vi "连接拧紧轴数据库.vi"(8 "error in (no error)":errorcluster, 9 "30":string="0", 10 "1":string="0", 11 "确定按钮":bool) -> (0 "error out":errorcluster, 1 "子数组":string[](array[string]), 2 "时间":string, 3 "索引结果":bool=TRUE)   [LabVIEW 2013]
uses:
  <vilib>/Utility/error.llb/whitespace.ctl
panel:
  out "error out 3":errorcluster
  out "error out 2":errorcluster
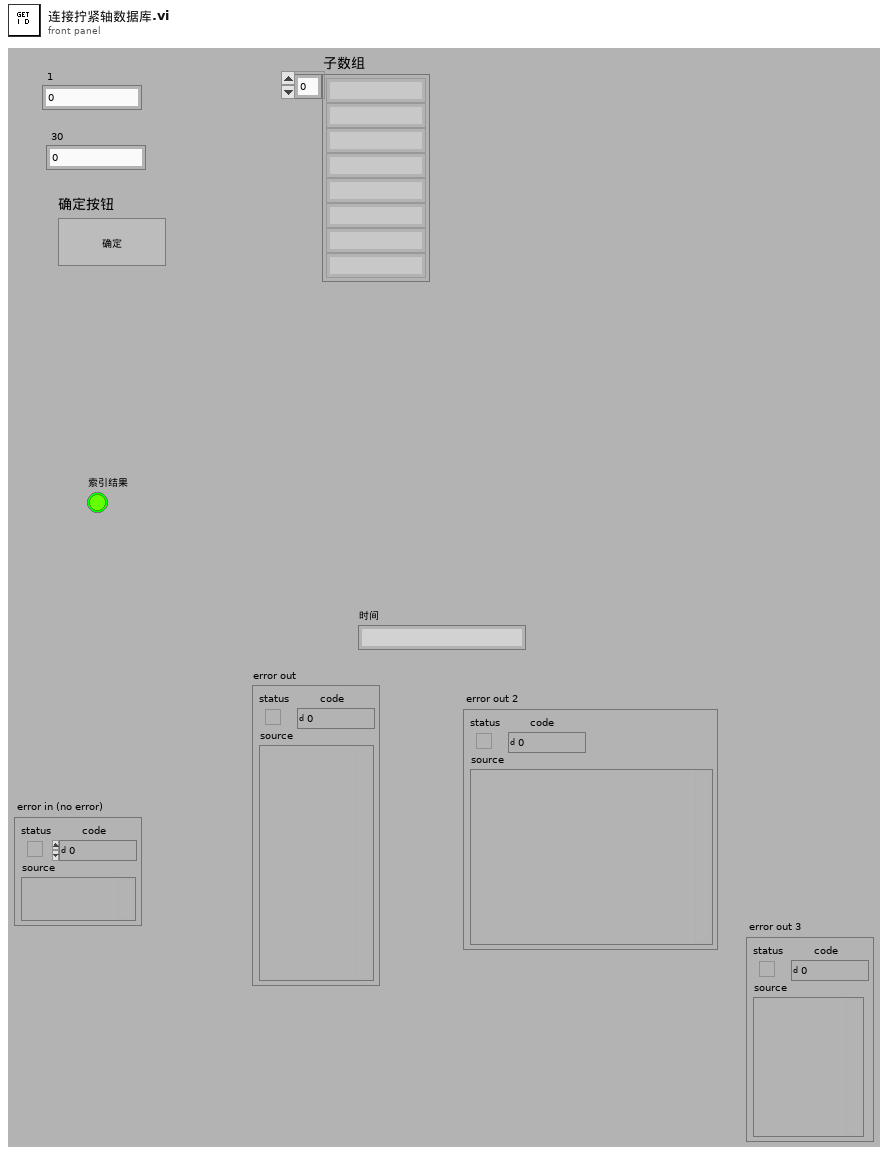
[diagram p1: front panel]
types:
  T1 = typedef "whitespace.ctl" = u16
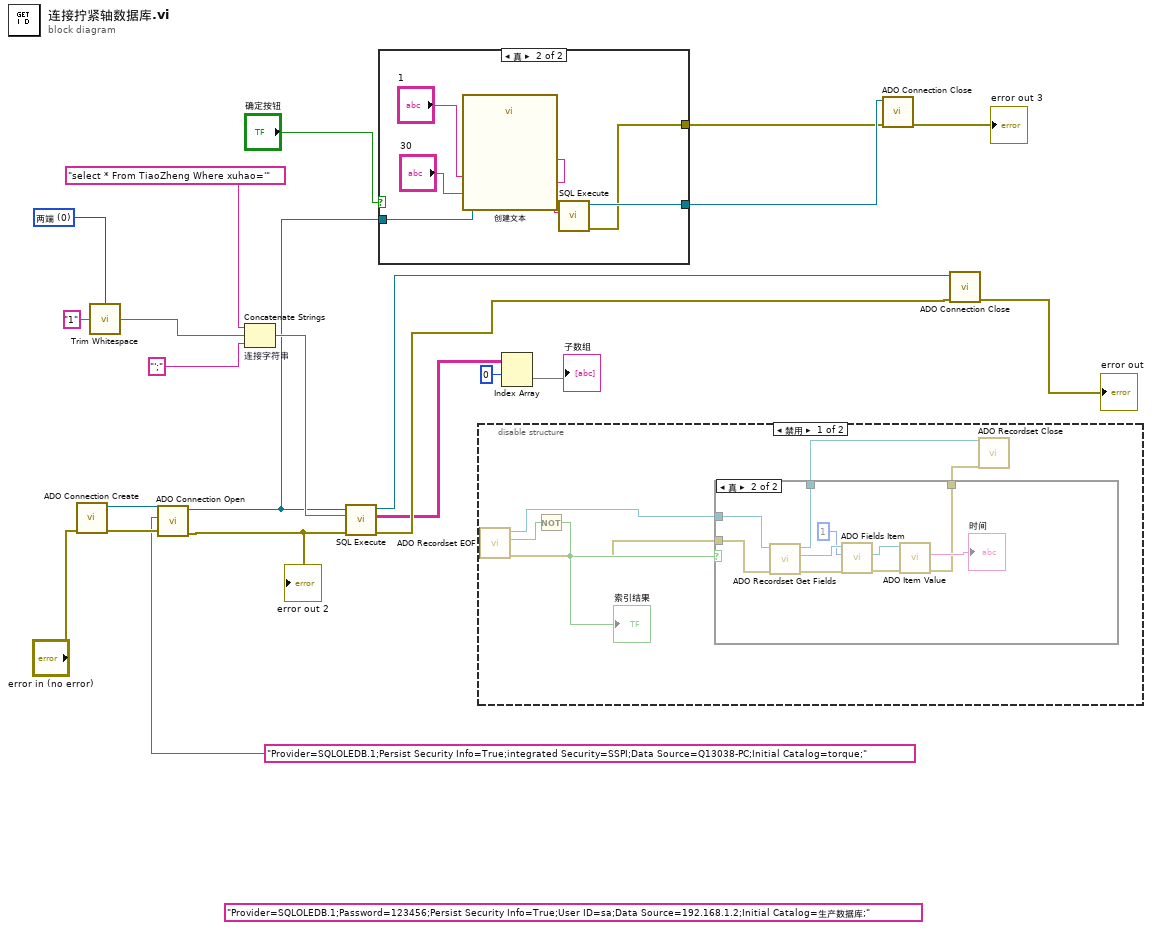
[diagram p0: block diagram]
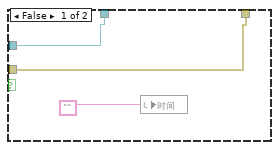
[diagram p3: hidden frame]
diagram:
  (unwired) "Provider=SQLOLEDB.1;Password=123456;Persist Security Info=True;User ID=sa;Data Source=192.168.1.2;Initial Catalog=生产数据库;" ("字符串 2")
  w15 = T1 0 items=["两端", "字符串首端", "字符串末端"] ("location (both)")
  n1 = call "ADO Connection Create.vi"("error in (no error)"="error in (no error)") -> ("error out"=w21:errorcluster, "ADODB._Connection Out"=w22:refnum<k7>)  [unwired: 9 out]
  n2 = call <vilib>:"Trim Whitespace.vi"("string"="1", "location (both)"=w15) -> ("trimmed string"=w16:string)
  n3 = call "ADO Connection Open.vi"("error in (no error)"=w21, "ConnectionString"="Provider=SQLOLEDB.1;Persist Security Info=True;integrated Security=SSPI;Data Source=Q13038-PC;Initial Catalog=torque;" ("字符串 2"), "ADODB._Connection In"=w22) -> ("error out"=w20:errorcluster, "ADODB._Connection Out"=w5:refnum<k7>)  [unwired: 7 out]
  "error out 2" <- w20
  n4 = Concatenate Strings "连接字符串"("select * From TiaoZheng Where xuhao='" ("字符串 2"), w16, "';" ("字符串 2")) -> (w6:string)
  n5 = call "SQL Execute.vi"("error in (no error)"=w20, "Command Text"=w6, "ADODB._Connection In"=w5) -> ("error out"=w10:errorcluster, "Data"=w9:string[][], "ADODB._Connection Out"=w11:refnum<k7>)  [unwired: 5 in, 1 out]
  n6 = case shown="真" "确定按钮" {
    tunnel: w5 -> [_ w28]
    tunnel: [_ w26] -> w3
    tunnel: [_ w23] -> w2
    frame False {
    }
    frame True {
      n7 = call "创建文本"("1"="1", "30"="30") -> ("Result"=w27:string)  [unwired: 12 in, 1 out]
      n8 = call "SQL Execute.vi"("Command Text"=w27, "ADODB._Connection In"=w28) -> ("error out"=w23:errorcluster, "ADODB._Connection Out"=w26:refnum<k7>)  [unwired: 6 in, 2 out]
    }
  }
  n9 = disable-structure shown="禁用" {
    frame Disabled {
      n10 = call "ADO Recordset EOF.vi"() -> ("error out"=w31:errorcluster, "EOF"=w34:bool, "ADODB._Recordset Out"=w32:refnum<k7>)  [unwired: 2 in, 7 out]
      n11 = Not(x=w34) -> (.not. x?=w33:bool)
      "索引结果" <- w33
      n12 = case shown="真" w33 {
        tunnel: w32 -> [w36 w47]
        tunnel: w31 -> [w37 w46]
        tunnel: [w36 w45] -> w30
        tunnel: [w37 w39] -> w29
        frame False {
          n13 = local write "时间"("") -> ()
        }
        frame True {
          n14 = call "ADO Recordset Get Fields.vi"("error in (no error)"=w46, "ADODB._Recordset In"=w47) -> ("error out"=w38:errorcluster, "Fields Out"=w44:refnum<k7>, "ADODB._Recordset Out"=w45:refnum<k7>)  [unwired: 7 out]
          n15 = call "ADO Fields Item.vi"("error in (no error)"=w38, "Index"=1, "Fields In"=w44) -> ("error out"=w42:errorcluster, "Item Out"=w41:refnum<k7>)  [unwired: 7 out]
          n16 = call "ADO Item Value.vi"("error in (no error)"=w42, "Item In"=w41) -> ("error out"=w39:errorcluster, "Value"=→"时间":string)  [unwired: 8 out]
        }
      }
      n17 = call "ADO Recordset Close.vi"("ADODB._Recordset In"=w30, "error in (no error)"=w29) -> ()  [unwired: 18 out]
    }
    frame Enabled {
    }
  }
  n18 = Index Array(array=w9, index (row)=0 ("索引 (行)")) -> (element=→"子数组":string[])  [unwired: 1 in]
  n19 = call "ADO Connection Close.vi"("error in (no error)"=w2, "ADODB._Connection In"=w3) -> ("error out"=→"error out 3":errorcluster)  [unwired: 9 out]
  n20 = call "ADO Connection Close.vi"("error in (no error)"=w10, "ADODB._Connection In"=w11) -> ("error out"=→"error out":errorcluster)  [unwired: 9 out]
